vi "State Size.vi"(8 "error in (no error)":errorcluster) -> (0 "error out":errorcluster, 2 "size":u64 format="%d bytes")   [LabVIEW 2019, in "DSF Core.lvlib" / "State.lvclass"]
uses:
  State.lvclass
  State Data.ctl
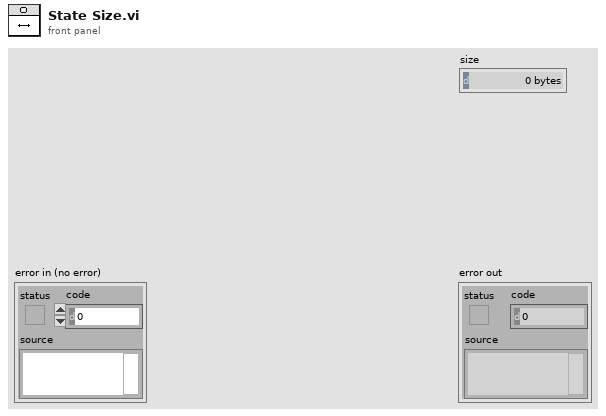
[diagram p1: front panel]
types:
  T1 = typedef "DSF Core.lvlib/State.lvclass/State Data.ctl" = cluster{"state":u8}
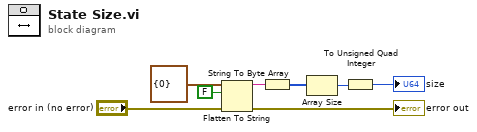
[diagram p0: block diagram]
diagram:
  n1 = Flatten To String(anything=T1 {"state"=0} ("state data"), prepend array or string size? (T)=FALSE, error in (no error)="error in (no error)") -> (data string=w5:string, error out=→"error out":errorcluster)  [unwired: 1 in, 1 out]
  n2 = String To Byte Array(string=w5) -> (unsigned byte array=w4:u8[])
  n3 = Array Size(array=w4) -> (size(s)=w2:i32)
  n4 = To Unsigned Quad Integer(1:w2) -> (0:→"size":u64)
